vi "fgv_Sys and HW Config.vi"(5 "Standalone viewer initialisation?":bool, 7 "Function":T19, 8 "error in (no error)":errorcluster, 10 "System Config":T1={"Laser wavelength (nm)"=920.0, "DAQ FPGA System"={"Clock Freq (MHz) "=200.0, "Samples Wait after Trigger"=5080, "AOD fill"=4900, "StartupDelay"=0, "Slip Cycle (clock cycles)"=600000, "Add Cycle"=TRUE}, "Control system"={"AOD 1 Amplitude"=0, "AOD 2 Amplitude"=0, "AOD 3 Amplitude"=0, "AOD 4 Amplitude"=0, "AOD 5 Amplitude"=0, "AOD 6 Amplitude"=0, "T0 (ns)"=0.0, "Ta (ns)"=0.0, "Data Time Interval (ns)"=0.0, "Ctrl FPGA Clock (MHz)"=240.0}} {"Control system"."Ctrl FPGA Clock (MHz)" min=80.0 max=500.0 step=1.0; "Control system"."Data Time Interval (ns)" min=0.0 max=2048.0 step=1.0; "Control system"."Ta (ns)" min=0.0 max=2048.0 step=1.0; "Control system"."T0 (ns)" min=0.0 max=2048.0 step=1.0; "Control system"."AOD 6 Amplitude" min=0 max=2048 step=1; "Control system"."AOD 5 Amplitude" min=0 max=2048 step=1; "Control system"."AOD 4 Amplitude" min=0 max=2048 step=1; "Control system"."AOD 3 Amplitude" min=0 max=2048 step=1; "Control system"."AOD 2 Amplitude" min=0 max=2048 step=1; "Control system"."AOD 1 Amplitude" min=0 max=2048 step=1; "Laser wavelength (nm)" min=800.0 max=1080.0 step=1.0}, 11 "Hardware Configuration":T4={"Dev. PC"=FALSE, "Swap XY on stage"=FALSE, "No of AOD"=0, "Computer MAC address"="", "Externalise Triggers"=FALSE, "Trigger HW config"={"Available Device List"=0, "Device Address"=""}, "DAQmx Chan"={"Pockels AO"="", "Hard shutter AO"="", "PMT AOs"="", "Galvo AOs"="", "Power meter AI"=""}, "XY stage available"=FALSE, "XY Stage"={"COM port"="", "Baudrate"=0, "Type"=""}, "Z stage available"=FALSE, "Z Stage config cluster"={"COM port"="COM7", "Baudrate"=0, "Type"=""}, "Encoder available"=FALSE, "Encoder"={"IP address"="224.0.1.103", "Port"=7000, "Wheel radius (cm)"=16.0, "Encoder Trigger"=""}, "VidRec available"=FALSE, "Cam VidRec"={"DO flag-Video record"="", "DO flag-Trial start"=""}, "Laser Power Control HW config"={"Laser Power Control"="", "Laser Power Modulation Control"=enum."NI"}, "Laser 1 available"=FALSE, "Laser 1 config cluster"={"COM port"="COM7", "Baud Rate"=0, "Type"=""}, "Prechirper 1 available"=FALSE, "Prechirper 1 config cluster"={"Type"="", "Baud Rate"=0, "COM port"="COM7"}, "Control system.FPGA available?"=FALSE, "Control Sys. HW config"={"Control system.FPGA Type"=enum."Virtex 5", "Control system.Network adapter name"="", "Control system.MAC address"="", "Control system.Ethernet Port"=0, "Control system.Ethernet Port Opened"=FALSE}, "DAQ FPGA HW Config"={"FGPA Ref"=refnum, "Target"="RIO0", "input card type"=enum."AC Card"}} {"Encoder"."Wheel radius (cm)" format="%#_13g"}) -> (0 "error out":errorcluster, 2 "System Config OUT":T1={"Laser wavelength (nm)"=920.0, "DAQ FPGA System"={"Clock Freq (MHz) "=200.0, "Samples Wait after Trigger"=5080, "AOD fill"=4900, "StartupDelay"=0, "Slip Cycle (clock cycles)"=600000, "Add Cycle"=TRUE}, "Control system"={"AOD 1 Amplitude"=0, "AOD 2 Amplitude"=0, "AOD 3 Amplitude"=0, "AOD 4 Amplitude"=0, "AOD 5 Amplitude"=0, "AOD 6 Amplitude"=0, "T0 (ns)"=0.0, "Ta (ns)"=0.0, "Data Time Interval (ns)"=0.0, "Ctrl FPGA Clock (MHz)"=240.0}} {"Control system"."Ctrl FPGA Clock (MHz)" min=80.0 max=500.0 step=1.0; "Control system"."Data Time Interval (ns)" min=0.0 max=2048.0 step=1.0; "Control system"."Ta (ns)" min=0.0 max=2048.0 step=1.0; "Control system"."T0 (ns)" min=0.0 max=2048.0 step=1.0; "Control system"."AOD 6 Amplitude" min=0 max=2048 step=1; "Control system"."AOD 5 Amplitude" min=0 max=2048 step=1; "Control system"."AOD 4 Amplitude" min=0 max=2048 step=1; "Control system"."AOD 3 Amplitude" min=0 max=2048 step=1; "Control system"."AOD 2 Amplitude" min=0 max=2048 step=1; "Control system"."AOD 1 Amplitude" min=0 max=2048 step=1; "Laser wavelength (nm)" min=800.0 max=1080.0 step=1.0}, 3 "Hardware Configuration OUT":T4={"Dev. PC"=FALSE, "Swap XY on stage"=FALSE, "No of AOD"=0, "Computer MAC address"="", "Externalise Triggers"=FALSE, "Trigger HW config"={"Available Device List"=0, "Device Address"=""}, "DAQmx Chan"={"Pockels AO"="", "Hard shutter AO"="", "PMT AOs"="", "Galvo AOs"="", "Power meter AI"=""}, "XY stage available"=FALSE, "XY Stage"={"COM port"="", "Baudrate"=0, "Type"=""}, "Z stage available"=FALSE, "Z Stage config cluster"={"COM port"="COM7", "Baudrate"=0, "Type"=""}, "Encoder available"=FALSE, "Encoder"={"IP address"="224.0.1.103", "Port"=7000, "Wheel radius (cm)"=16.0, "Encoder Trigger"=""}, "VidRec available"=FALSE, "Cam VidRec"={"DO flag-Video record"="", "DO flag-Trial start"=""}, "Laser Power Control HW config"={"Laser Power Control"="", "Laser Power Modulation Control"=enum."NI"}, "Laser 1 available"=FALSE, "Laser 1 config cluster"={"COM port"="COM7", "Baud Rate"=0, "Type"=""}, "Prechirper 1 available"=FALSE, "Prechirper 1 config cluster"={"Type"="", "Baud Rate"=0, "COM port"="COM7"}, "Control system.FPGA available?"=FALSE, "Control Sys. HW config"={"Control system.FPGA Type"=enum."Virtex 5", "Control system.Network adapter name"="", "Control system.MAC address"="", "Control system.Ethernet Port"=0, "Control system.Ethernet Port Opened"=FALSE}, "DAQ FPGA HW Config"={"FGPA Ref"=refnum, "Target"="RIO0", "input card type"=enum."AC Card"}} {"Encoder"."Wheel radius (cm)" format="%#_13g"})   [LabVIEW 2017]
uses:
  Typedefs/HW config states enum.ctl
  Typedefs/System Configuration.ctl
  Typedefs/DAQ FPGA system config.ctl
  Typedefs/CTRL system config.ctl
  Typedefs/Hardware Configuration settings.ctl
  Typedefs/Triggers HW config.ctl
  Typedefs/DAQmx physical channels cluster.ctl
  Typedefs/XY Stage config cluster.ctl
  Typedefs/Z Stage config cluster.ctl
  Typedefs/Encoder config cluster.ctl
  Typedefs/Cam VidRec HW config setup cluster.ctl
  Typedefs/Laser Power Control HW config.ctl
  Typedefs/Laser 1 config cluster.ctl
  Typedefs/PreChirper 1 config cluster.ctl
  Typedefs/Control Sys HW config cluster.ctl
  Typedefs/DAQ FPGA HW config cluster.ctl
  RIG-SPECIFIC FILES/FPGA Refs/FPGA Ref.ctl
  <vilib>/userdefined/High Color/nirio_resource_hc.ctl
  Typedefs/FPGA input type AC-DC.ctl
  Typedefs/Save-Load enum.ctl
  General Globals.vi
panel:
  # "FUNCTIONAL GLOBAL"
  # "<--- The \"PMT AOs\" DAQmx string will always contain\n                       2 channels is this format: PXI1Slot4/ao2:3"
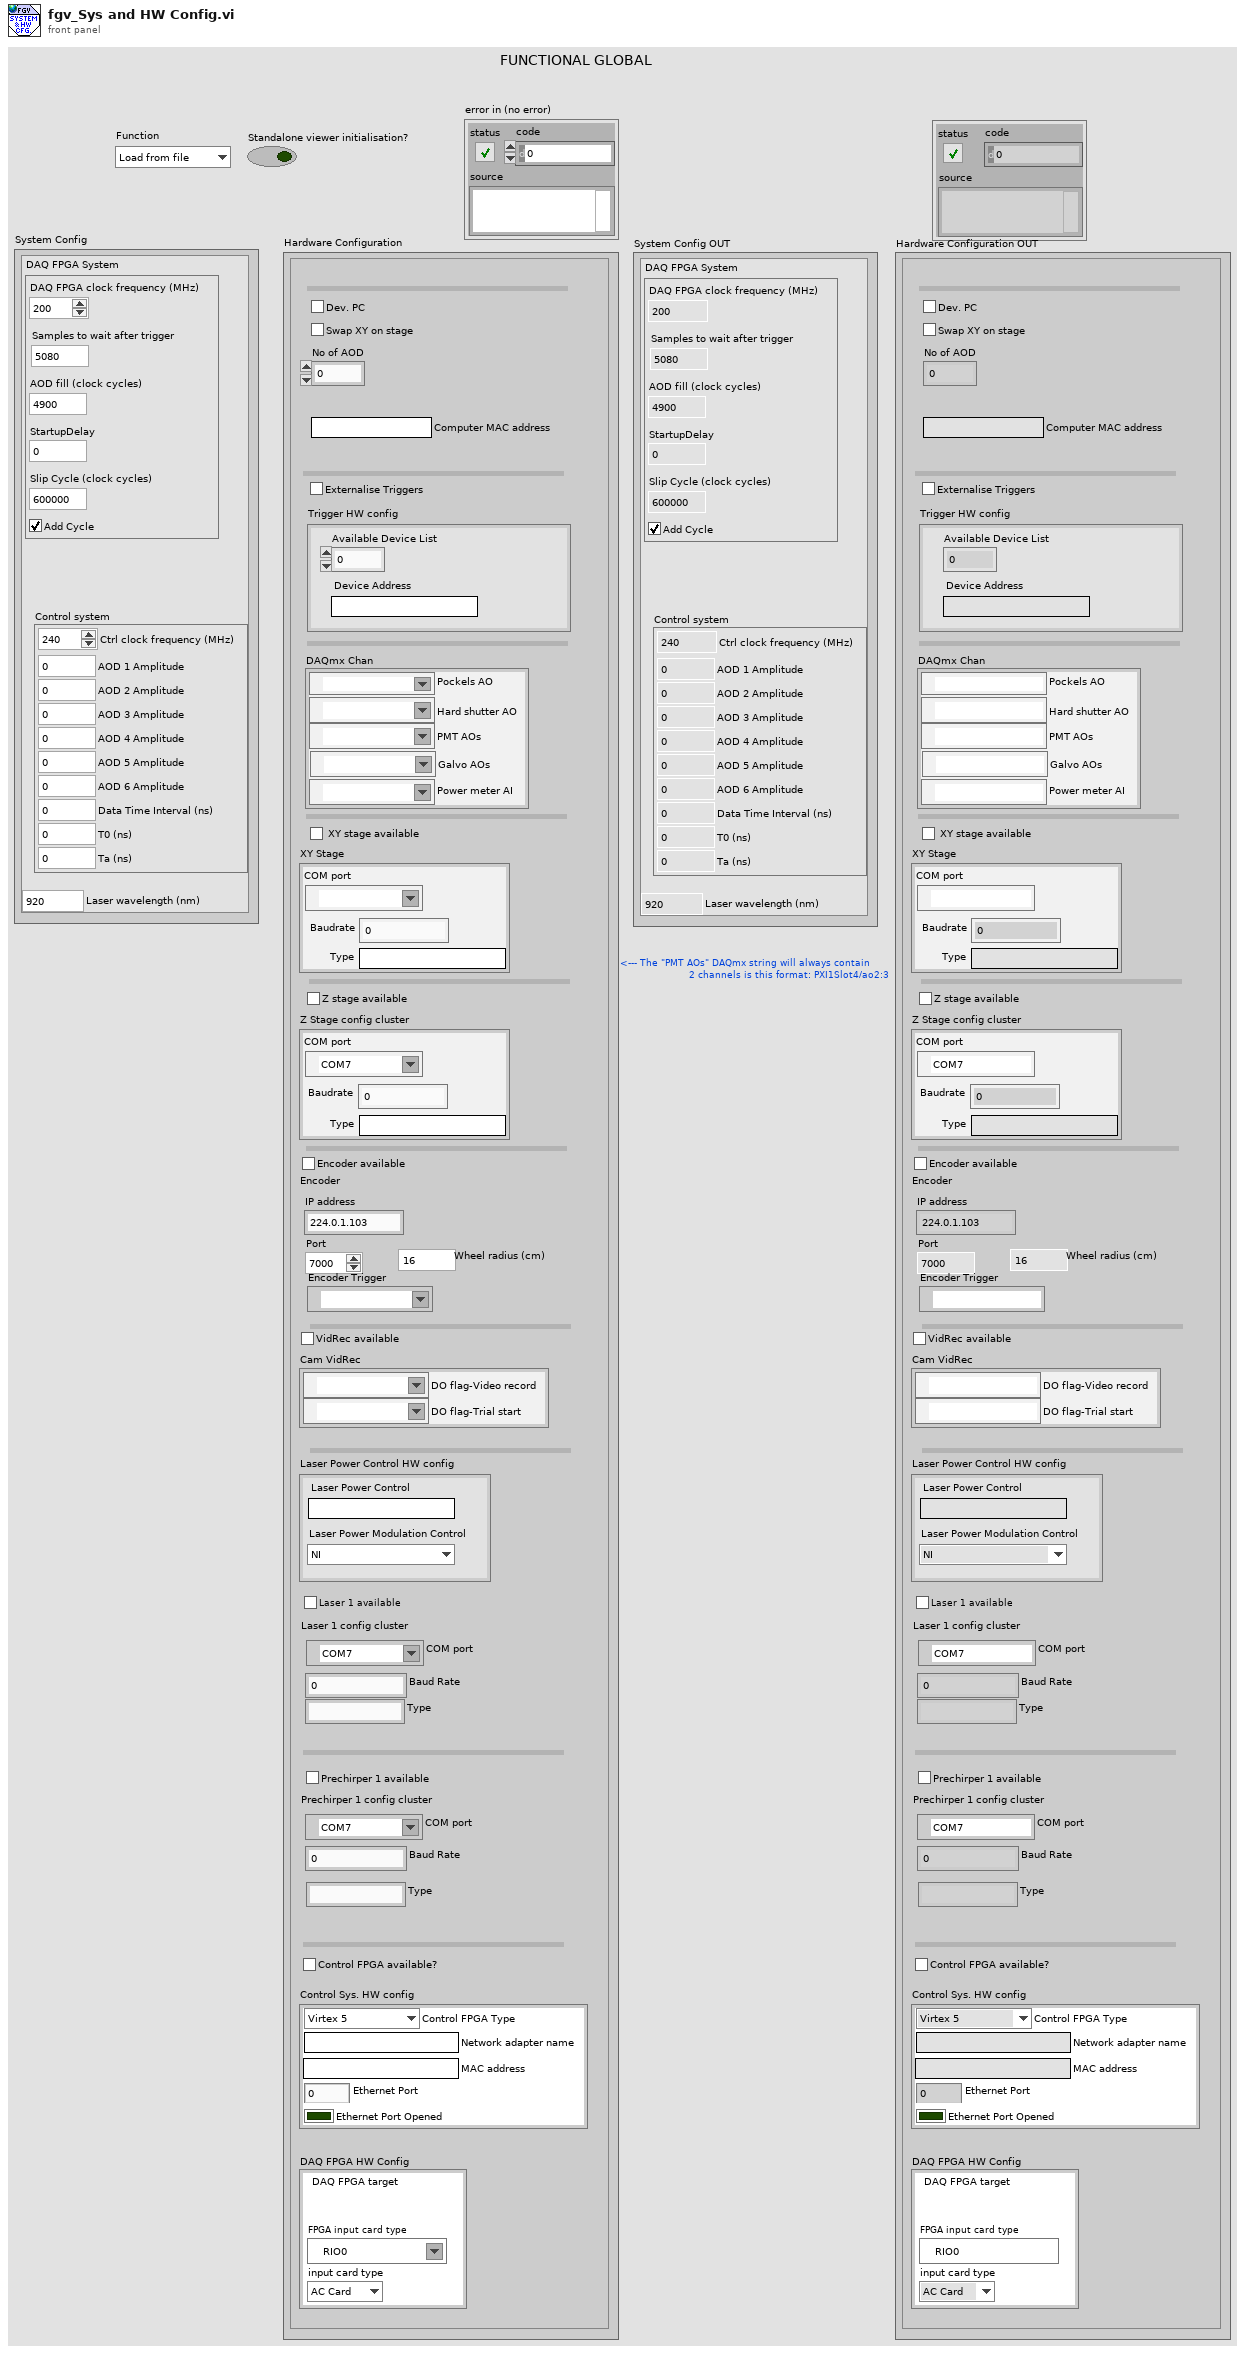
[diagram p1: front panel]
types:
  T1 = typedef "System Configuration.ctl" = cluster{"Laser wavelength (nm)":dbl, "DAQ FPGA System":T2, "Control system":T3}
  T2 = typedef "DAQ FPGA system config.ctl" = cluster{"Clock Freq (MHz) ":dbl, "Samples Wait after Trigger":u16, "AOD fill":u16, "StartupDelay":i32, "Slip Cycle (clock cycles)":u32, "Add Cycle":bool}
  T3 = typedef "CTRL system config.ctl" = cluster{"AOD 1 Amplitude":i16, "AOD 2 Amplitude":i16, "AOD 3 Amplitude":i16, "AOD 4 Amplitude":i16, "AOD 5 Amplitude":i16, "AOD 6 Amplitude":i16, "T0 (ns)":dbl, "Ta (ns)":dbl, "Data Time Interval (ns)":dbl, "Ctrl FPGA Clock (MHz)":dbl}
  T4 = typedef "Hardware Configuration settings.ctl" = cluster{"Dev. PC":bool, "Swap XY on stage":bool, "No of AOD":u8, "Computer MAC address":string, "Externalise Triggers":bool, "Trigger HW config":T5, "DAQmx Chan":T6, "XY stage available":bool, "XY Stage":T7, "Z stage available":bool, "Z Stage config cluster":T8, "Encoder available":bool, "Encoder":T9, "VidRec available":bool, "Cam VidRec":T10, "Laser Power Control HW config":T11, "Laser 1 available":bool, "Laser 1 config cluster":T12, "Prechirper 1 available":bool, "Prechirper 1 config cluster":T13, "Control system.FPGA available?":bool, "Control Sys. HW config":T14, "DAQ FPGA HW Config":T15}
  T5 = typedef "Triggers HW config.ctl" = cluster{"Available Device List":i32, "Device Address":string}
  T6 = typedef "DAQmx physical channels cluster.ctl" = cluster{"Pockels AO":tag, "Hard shutter AO":tag, "PMT AOs":tag, "Galvo AOs":tag, "Power meter AI":tag}
  T7 = typedef "XY Stage config cluster.ctl" = cluster{"COM port":refnum<visa-resource-name>, "Baudrate":i32, "Type":string}
  T8 = typedef "Z Stage config cluster.ctl" = cluster{"COM port":refnum<visa-resource-name>, "Baudrate":i32, "Type":string}
  T9 = typedef "Encoder config cluster.ctl" = cluster{"IP address":string, "Port":u16, "Wheel radius (cm)":dbl, "Encoder Trigger":tag}
  T10 = typedef "Cam VidRec HW config setup cluster.ctl" = cluster{"DO flag-Video record":tag, "DO flag-Trial start":tag}
  T11 = typedef "Laser Power Control HW config.ctl" = cluster{"Laser Power Control":string, "Laser Power Modulation Control":enum16{"NI", "FPGA"}}
  T12 = typedef "Laser 1 config cluster.ctl" = cluster{"COM port":refnum<visa-resource-name>, "Baud Rate":i32, "Type":string}
  T13 = typedef "PreChirper 1 config cluster.ctl" = cluster{"Type":string, "Baud Rate":i32, "COM port":refnum<visa-resource-name>}
  T14 = typedef "Control Sys HW config cluster.ctl" = cluster{"Control system.FPGA Type":enum16{"Virtex 5", "Virtex 7"}, "Control system.Network adapter name":string, "Control system.MAC address":string, "Control system.Ethernet Port":u32, "Control system.Ethernet Port Opened":bool}
  T15 = typedef "DAQ FPGA HW config cluster.ctl" = cluster{"FGPA Ref":T16, "Target":T17, "input card type":T18}
  T16 = typedef "FPGA Ref.ctl" = refnum<k20>
  T17 = typedef "nirio_resource_hc.ctl" = tag
  T18 = typedef "FPGA input type AC-DC.ctl" = enum16{"AC Card", "DC Card"}
  T19 = typedef "HW config states enum.ctl" = enum16{"Load from file", "Save to file", "Write all", "Read all", "Write XY stage settings", "Write DAQ FPGA settings", "Write Control FPGA settings", "Write Phys Channels", "Write System Config", "Write HW Config", "Save System Config", "Save HW Config", "Clear", "Compare from file"}
  T20 = typedef "Save-Load enum.ctl" = enum16{"Save to file", "Load from file", "Compare from file"}
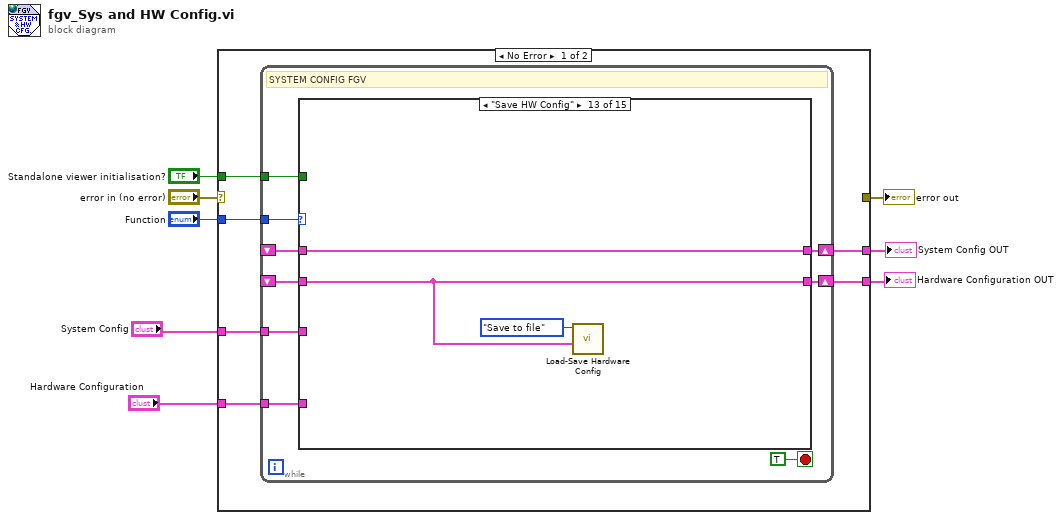
[diagram p0: block diagram]
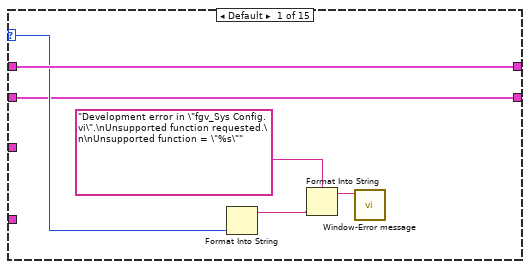
[diagram p2: hidden frame]
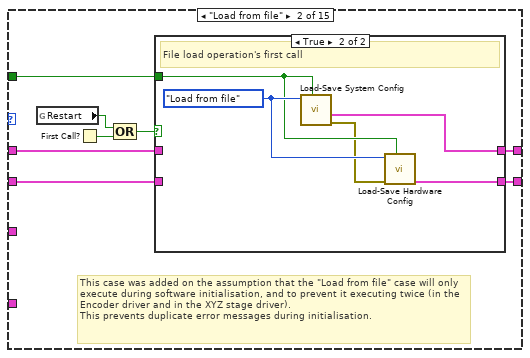
[diagram p3: hidden frame]
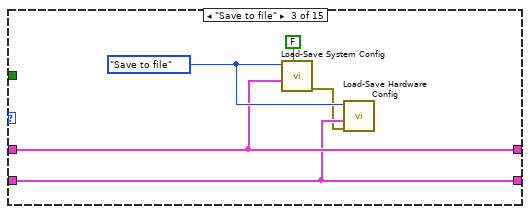
[diagram p5: hidden frame]
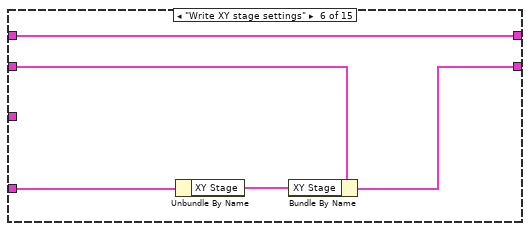
[diagram p8: hidden frame]
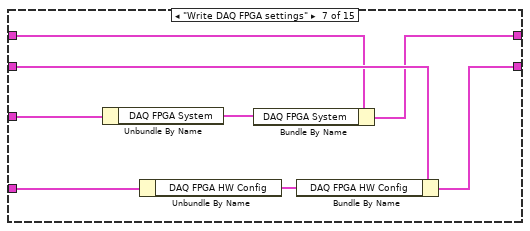
[diagram p9: hidden frame]
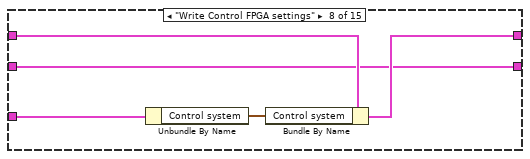
[diagram p10: hidden frame]
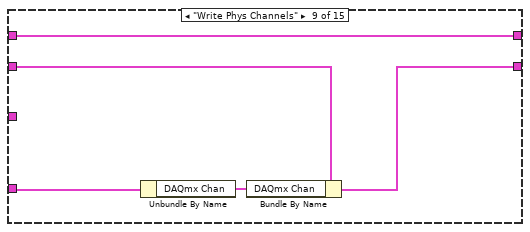
[diagram p11: hidden frame]
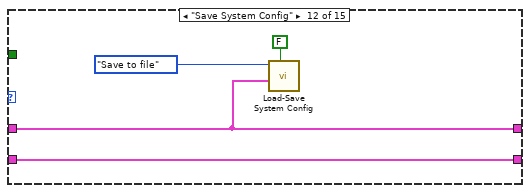
[diagram p14: hidden frame]
diagram:
  n1 = case shown="No Error" "error in (no error)" {
    selector: "error in (no error)" -> [_ w90]
    tunnel: [_ w90] -> w7
    tunnel: "Function" -> [w14 _]
    tunnel: "System Config" -> [w13 _]
    tunnel: [w12 _] -> w1
    tunnel: "Standalone viewer initialisation?" -> [w11 _]
    tunnel: "Hardware Configuration" -> [w10 _]
    tunnel: [w9 _] -> w2
    frame No Error {
      n2 = while {
        tunnel: w14 -> [w23]
        shift-right: [w21] -> w12
        shift-left: _ -> [w19]
        tunnel: w13 -> [w20]
        tunnel: w11 -> [w18]
        tunnel: w10 -> [w17]
        shift-right: [w16] -> w9
        shift-left: _ -> [w15]
        stop <- TRUE stop-if-true
        # "SYSTEM CONFIG FGV"
        n3 = case shown="\"Save HW Config\"" w23 {
          selector: w23 -> [w25 _ _ _ _ _ _ _ _ _ _ _ _ _ _]
          tunnel: [w26 w32 w47 w51 w53 w54 w60 w68 w75 w77 w80 w81 w87 w89 _] -> w21
          tunnel: w20 -> [_ _ _ w51 _ _ w62 w71 _ w77 _ _ _ _ _]
          tunnel: w19 -> [w26 w37 w47 _ w53 w54 w61 w70 w75 _ w80 w81 w87 w89 _]
          tunnel: w18 -> [_ w33 _ _ _ _ _ _ _ _ _ _ _ _ _]
          tunnel: w17 -> [_ _ _ w50 _ w57 w65 _ w74 _ w79 _ _ _ _]
          tunnel: [w24 w31 w46 w50 w52 w55 w63 w67 w72 w78 w79 w84 w85 w88 _] -> w16
          tunnel: w15 -> [w24 w30 w46 _ w52 w56 w64 w67 w73 w78 _ w84 w85 w88 _]
          frame Default {
            n4 = Format Into String(w25) -> (resulting string=w28:string)  [unwired: 3 in, 1 out]
            n5 = Format Into String(format string="Development error in \"fgv_Sys Config.vi\".\nUnsupported function requested.\n\nUnsupported function = \"%s\"" ("Message"), w28) -> (resulting string=w27:string)  [unwired: 2 in, 1 out]
            n6 = call "Window-Error message.vi"("Message"=w27) -> ()  [unwired: 10 in, 1 out]
          }
          frame "Load from file" {
            # "This case was added on the assumption that the \"Load from file\" case will only execute during software initialisation, and to prevent it executing twice (in the Encoder driver and in the XYZ stage driver).\nThis prevents duplicate error messages during initialisation."
            n7 = global read "General Globals.vi" "Restart"() -> (w34:bool)
            n8 = First Call?() -> (First Call?: T/F=w36:bool)
            n9 = Compound Arithmetic op=OR(w34, w36) -> (w35:bool)
            n10 = case shown="True" w35 {
              tunnel: w37 -> [w39 _]
              tunnel: w33 -> [_ w41]
              tunnel: [w39 w44] -> w32
              tunnel: [w38 w42] -> w31
              tunnel: w30 -> [w38 _]
              frame False {
                # "Already loaded"
              }
              frame True {
                w43 = Save-Load_enum."Load from file" ("Function")
                # "File load operation's first call"
                n11 = call "Load-Save System Config.vi"("Standalone viewer?"=w41, "Function"=w43) -> ("error out"=w40:errorcluster, "System Config O/P"=w44:T1)  [unwired: 8 in]
                n12 = call "Load-Save Hardware Config.vi"("Standalone ?"=w41, "error in"=w40, "Function"=w43) -> ("Hardware Configuration O/P"=w42:T4)  [unwired: 7 in, 1 out]
              }
            }
          }
          frame "Save to file" {
            w48 = Save-Load_enum."Save to file" ("Function")
            n13 = call "Load-Save System Config.vi"("Standalone viewer?"=FALSE, "System Config I/P"=w47, "Function"=w48) -> ("error out"=w45:errorcluster)  [unwired: 7 in, 1 out]
            n14 = call "Load-Save Hardware Config.vi"("error in"=w45, "Hardware Configuration I/P"=w46, "Function"=w48) -> ()  [unwired: 7 in, 2 out]
          }
          frame "Write all" {
          }
          frame "Read all" {
          }
          frame "Write XY stage settings" {
            n15 = Unbundle By Name(w57) -> ("XY Stage"=w58:T7)
            n16 = Bundle By Name(cluster=w56, "XY Stage"=w58) -> (w55:T4)
          }
          frame "Write DAQ FPGA settings" {
            n17 = Unbundle By Name(w62) -> ("DAQ FPGA System"=w59:T2)
            n18 = Unbundle By Name(w65) -> ("DAQ FPGA HW Config"=w66:T15)
            n19 = Bundle By Name(cluster=w61, "DAQ FPGA System"=w59) -> (w60:T1)
            n20 = Bundle By Name(cluster=w64, "DAQ FPGA HW Config"=w66) -> (w63:T4)
          }
          frame "Write Control FPGA settings" {
            n21 = Unbundle By Name(w71) -> ("Control system"=w69:T3)
            n22 = Bundle By Name(cluster=w70, "Control system"=w69) -> (w68:T1)
          }
          frame "Write Phys Channels" {
            n23 = Unbundle By Name(w74) -> ("DAQmx Chan"=w76:T6)
            n24 = Bundle By Name(cluster=w73, "DAQmx Chan"=w76) -> (w72:T4)
          }
          frame "Write System Config" {
          }
          frame "Write HW Config" {
          }
          frame "Save System Config" {
            n25 = call "Load-Save System Config.vi"("Standalone viewer?"=FALSE, "System Config I/P"=w81, "Function"=Save-Load_enum."Save to file") -> ()  [unwired: 7 in, 2 out]
          }
          frame "Save HW Config" {
            n26 = call "Load-Save Hardware Config.vi"("Hardware Configuration I/P"=w85, "Function"=Save-Load_enum."Save to file") -> ()  [unwired: 8 in, 2 out]
          }
          frame "Compare from file" {
          }
          frame "Clear" {
          }
        }
      }
    }
    frame Error {
    }
  }
  "error out" <- w7
  "Hardware Configuration OUT" <- w2
  "System Config OUT" <- w1
